vi "Puzzle 14-1.vi"() -> ()   [LabVIEW 2022 SP3]
panel:
  in  "delimited string":string="O....#....\nO.OO#....#\n.....##...\nOO.#O....O\n.O.....O#.\nO.#..O.#.#\n..O..#O..O\n.......O..\n#....###..\n#OO..#...."
  out "sum":i32
  out "unsigned byte array 2":u8[][](array[numeric])
  out "unsigned byte array":u8[][](array[numeric])
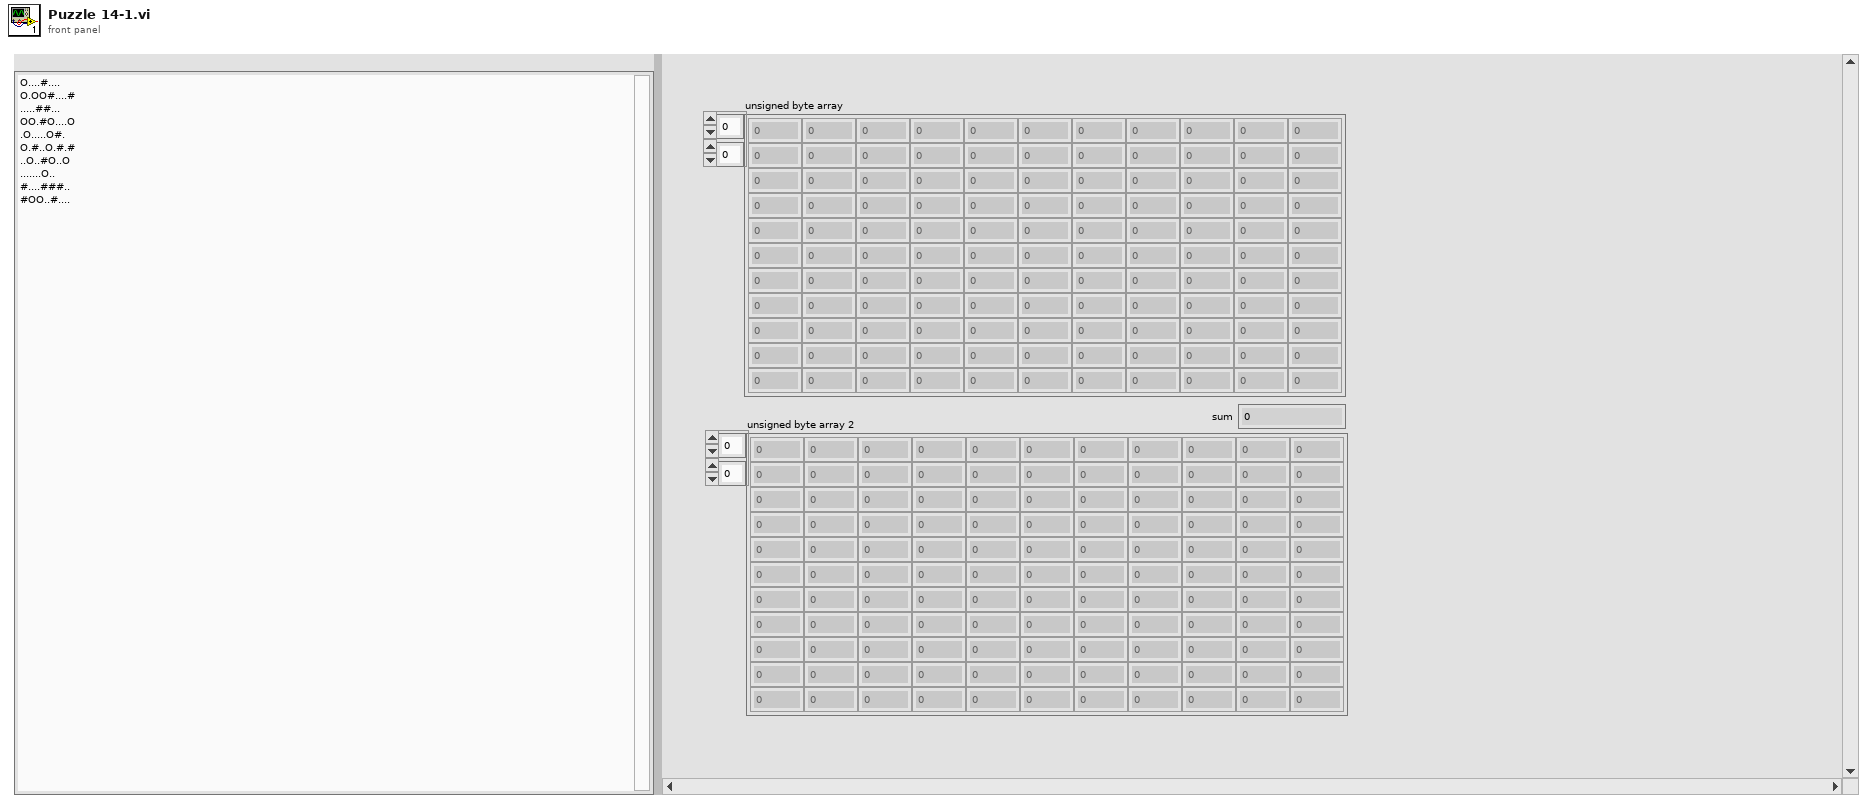
[diagram p1: front panel]
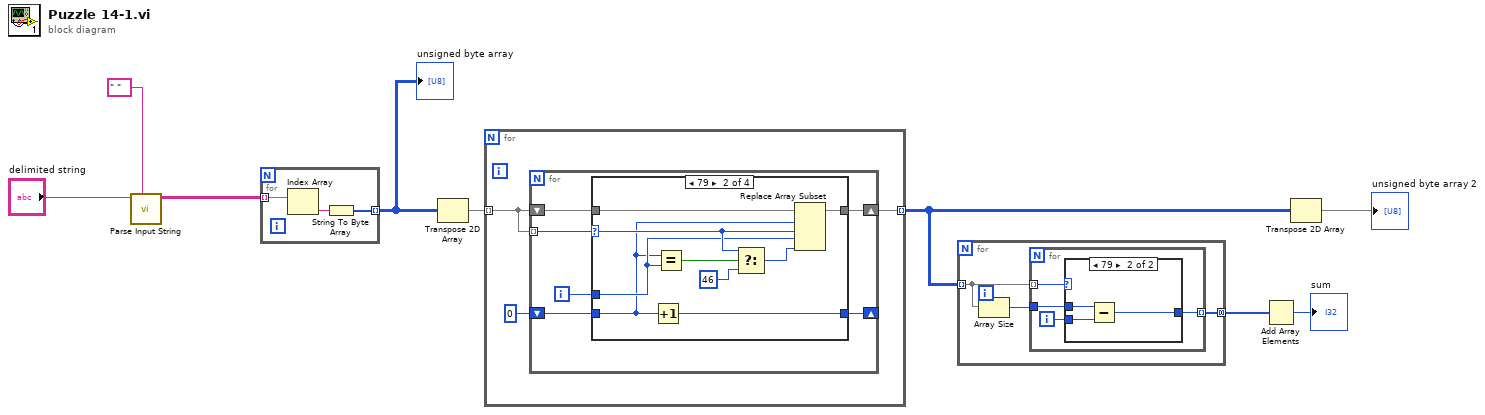
[diagram p0: block diagram]
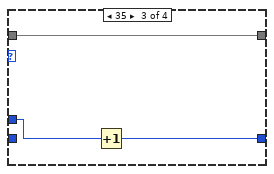
[diagram p4: hidden frame]
diagram:
  n1 = call "Parse Input String.vi"("delimiter (Tab)"=" ", "delimited string"="delimited string") -> ("parsed string"=w7:string[][])  [unwired: 9 in]
  n2 = for {
    tunnel: w7 -> [w12] mode=indexing
    tunnel: [w10] -> w6 mode=indexing
    n3 = Index Array(array=w12) -> (element=w11:string)  [unwired: 1 in]
    n4 = String To Byte Array(string=w11) -> (unsigned byte array=w10:u8[])
  }
  "unsigned byte array" <- w6
  n5 = Transpose 2D Array(2D array=w6) -> (transposed array=w5:u8[][])
  n6 = for {
    tunnel: w5 -> [w14] mode=indexing
    tunnel: [w13] -> w3 mode=indexing
    n7 = for {
      tunnel: w14 -> [w21] mode=indexing
      shift-right: [w19] -> _
      shift-left: 0 -> [w20]
      shift-right: [w17] -> w13
      shift-left: w14 -> [w18]
      i -> [w16]
      n8 = case shown="79" w21 {
        selector: w21 -> [_ w28 _ _]
        tunnel: w20 -> [w22 w24 _ w37]
        tunnel: [w22 w32 w34 w37] -> w19
        tunnel: w18 -> [w23 w31 w35 w36]
        tunnel: [w23 w30 w35 w36] -> w17
        tunnel: w16 -> [_ w25 w33 _]
        frame Default {
        }
        frame 79 {
          n9 = Increment(x=w24) -> (x+1=w32:i32)
          n10 = Equal?(x=w24, y=w25) -> (x = y?=w29:bool)
          n11 = Select(t=w28, s=w29, f=u8 46) -> (s? t:f=w26:u8)
          n12 = Replace Array Subset(array=w31, new element #1=w28, index #1=w24, new element #2=w26, index #2=w25) -> (w30:u8[])
        }
        frame 35 {
          n13 = Increment(x=w33) -> (x+1=w34:i32)
        }
        frame 46 {
        }
      }
    }
  }
  n14 = for {
    tunnel: w3 -> [w40] mode=indexing
    tunnel: [w38] -> w2 mode=concatenating
    n15 = Array Size(array=w40) -> (size(s)=w39:i32)
    n16 = for {
      tunnel: w40 -> [w44] mode=indexing
      tunnel: w39 -> [w43]
      tunnel: [w41] -> w38 mode=indexing
      i -> [w42]
      n17 = case shown="79" w44 {
        tunnel: w43 -> [_ w47]
        tunnel: w42 -> [_ w46]
        tunnel: [_ w45] -> w41
        frame Default {
        }
        frame 79 {
          n18 = Subtract(x=w47, y=w46) -> (x-y=w45:i32)
        }
      }
    }
  }
  n19 = Add Array Elements(numeric array=w2) -> (sum=→"sum":i32)
  n20 = Transpose 2D Array(2D array=w3) -> (transposed array=→"unsigned byte array 2":u8[][])
